vi "Write error cluster.vi"(8 "error in (no error)":errorcluster, 10 "error":errorcluster, 11 "Abstract Instrument in":refnum<class "Abstract Instrument.lvclass">) -> (0 "error out":errorcluster, 3 "Abstract Instrument out":refnum<class "Abstract Instrument.lvclass">)   [LabVIEW 2025, in "Abstract Engine.lvlib" / "Abstract Instrument.lvclass"]
uses:
  Abstract Instrument.lvclass
  Abstract Instrument.lvclass/Abstract Instrument.ctl
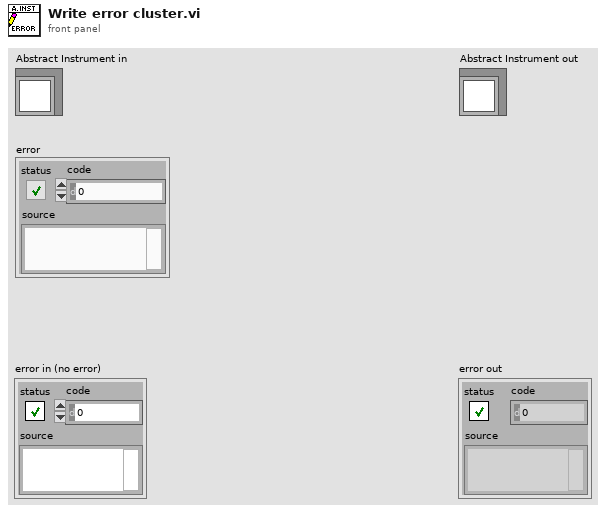
[diagram p1: front panel]
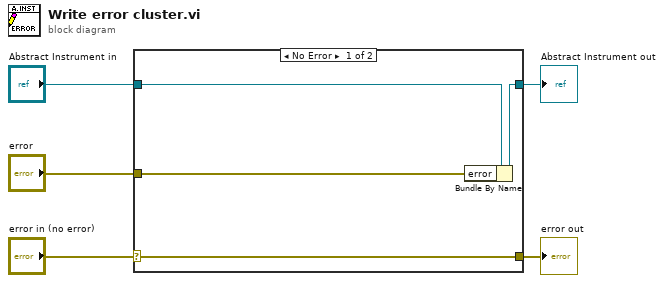
[diagram p0: block diagram]
diagram:
  n1 = case shown="No Error" "error in (no error)" {
    selector: "error in (no error)" -> [w9 w10]
    tunnel: [w9 w10] -> w4
    tunnel: [w7 w11] -> w2
    tunnel: "Abstract Instrument in" -> [w8 w11]
    tunnel: "error" -> [w6 _]
    frame No Error {
      n2 = Bundle By Name(cluster=w8, "error"=w6) -> (w7:refnum<class "Abstract Instrument.lvclass">)
    }
    frame Error {
    }
  }
  "error out" <- w4
  "Abstract Instrument out" <- w2
